vi "Actuator Channel Names DAO.vi"(5 "section":string="Auto Balance Error", 7 "Config Ref  In":T3, 8 "error in (no error)":errorcluster, 9 "Names In":T2, 10 "LBCB Number":T1, 11 "Actions":T4) -> (0 "error out":errorcluster, 1 "Names Out":T2, 6 "Config Ref Out":T3)   [LabVIEW 2009]
uses:
  Metadata/Persistant DAO Actions.ctl
  Metadata/Actuator Channel Names.ctl
  <vilib>/Utility/config.llb/Config Data RefNum.ctl
  Metadata/LBCB Number.ctl
  <vilib>/Utility/config.llb/NI_LVConfig.lvlib
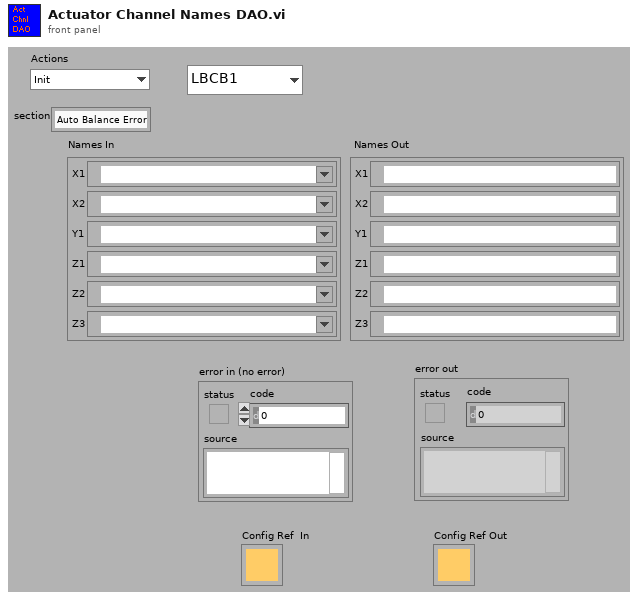
[diagram p1: front panel]
types:
  T1 = typedef "LBCB Number.ctl" = enum16{"LBCB1", "LBCB2"}
  T2 = typedef "Actuator Channel Names.ctl" = cluster{"X1":refnum<k21>, "X2":refnum<k21>, "Y1":refnum<k21>, "Z1":refnum<k21>, "Z2":refnum<k21>, "Z3":refnum<k21>}
  T3 = typedef "NI_LVConfig.lvlib/Config Data RefNum.ctl" = refnum<k1>
  T4 = typedef "Persistant DAO Actions.ctl" = enum16{"Init", "Get", "Set", "Load", "Save"}
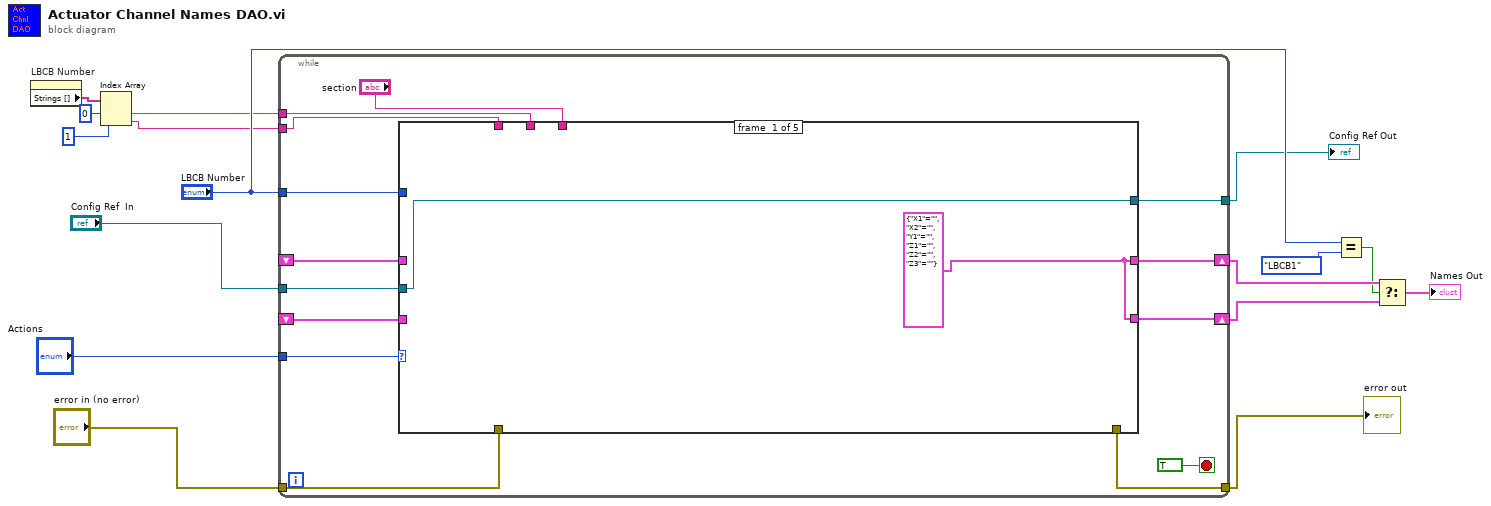
[diagram p0: block diagram]
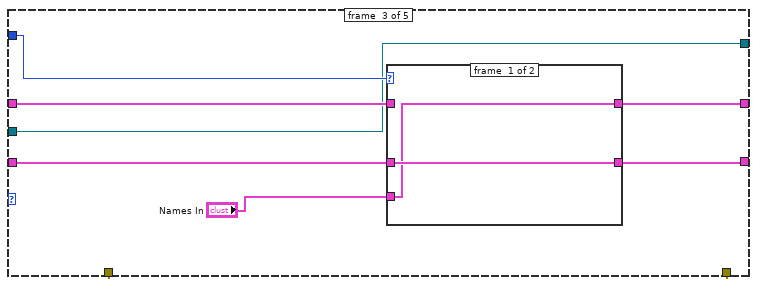
[diagram p3: hidden frame]
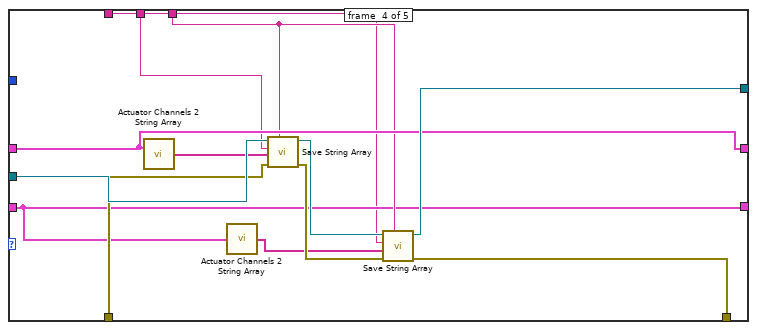
[diagram p5: hidden frame]
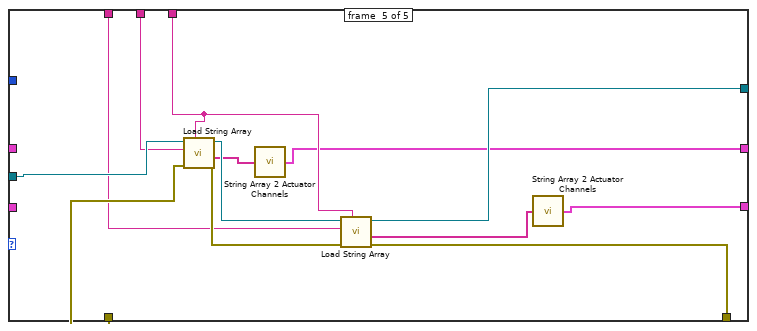
[diagram p6: hidden frame]
diagram:
  n1 = property on="LBCB Number" class="Enum (strict)"() -> ("Strings []"=w5:string[])  [unwired: 2 in, 2 out]
  n2 = Index Array(array=w5, index #1=0 ("index"), index #2=1 ("index")) -> (element #1=w2:string, element #2=w1:string)
  n3 = while {
    tunnel: "Actions" -> [w29]
    tunnel: "Config Ref  In" -> [w28]
    tunnel: "error in (no error)" -> [w26]
    tunnel: [w25] -> w6
    tunnel: [w24] -> w7
    shift-right: [w23] -> w13
    shift-left: _ -> [w22]
    tunnel: "LBCB Number" -> [w21]
    shift-right: [w20] -> w12
    shift-left: _ -> [w19]
    tunnel: w2 -> [w18]
    tunnel: w1 -> [w17]
    stop <- TRUE stop-if-true
    n4 = case shown="\"Load\"" w29 {
      tunnel: "section" -> [_ _ _ w54 w69]
      tunnel: w28 -> [w33 w35 w39 w62 w75]
      tunnel: w26 -> [w32 w34 w38 w61 w74]
      tunnel: [w33 w35 w39 w58 w71] -> w25
      tunnel: [w32 w34 w38 w57 w70] -> w24
      tunnel: [w31 w37 w40 w56 w63] -> w23
      tunnel: w22 -> [_ w37 w44 w56 _]
      tunnel: w21 -> [_ _ w45 _ _]
      tunnel: [w31 w36 w41 w53 w65] -> w20
      tunnel: w19 -> [_ w36 w43 w53 _]
      tunnel: w18 -> [_ _ _ w51 w68]
      tunnel: w17 -> [_ _ _ w50 w67]
      frame #0 {
        w31 = T2 {"X1"="", "X2"="", "Y1"="", "Z1"="", "Z2"="", "Z3"=""} ("Names In")
        (unwired) T2 {"X1"="", "X2"="", "Y1"="", "Z1"="", "Z2"="", "Z3"=""} ("Names In")
      }
      frame #1 {
      }
      frame #2 {
        n5 = case shown="\"LBCB2\"" w45 {
          tunnel: w44 -> [_ w49]
          tunnel: w43 -> [w47 _]
          tunnel: "Names In" -> [w46 w48]
          tunnel: [w46 w49] -> w40
          tunnel: [w47 w48] -> w41
          frame #0 {
          }
          frame #1 {
          }
        }
      }
      frame #3 {
        n6 = call "Actuator Channels 2 String Array.vi"("Actuator Channels"=w56) -> ("Array"=w55:string[])
        n7 = call "Actuator Channels 2 String Array.vi"("Actuator Channels"=w53) -> ("Array"=w52:string[])
        n8 = call "Save String Array.vi"("section"=w54, "error in (no error)"=w61, "String Array In"=w55, "key"=w51, "refnum"=w62) -> ("error out"=w60:errorcluster, "refnum out"=w59:T3)  [unwired: 1 in, 4 out]
        n9 = call "Save String Array.vi"("section"=w54, "error in (no error)"=w60, "String Array In"=w52, "key"=w50, "refnum"=w59) -> ("error out"=w57:errorcluster, "refnum out"=w58:T3)  [unwired: 1 in, 4 out]
      }
      frame #4 {
        n10 = call "Load String Array.vi"("section"=w69, "error in (no error)"=w74, "key"=w68, "refnum"=w75) -> ("error out"=w72:errorcluster, "String Array Out"=w64:string[], "refnum out"=w73:T3)  [unwired: 5 out]
        n11 = call "String Array 2 Actuator Channels.vi"("Array"=w64) -> ("Actuator Point"=w63:T2)
        n12 = call "Load String Array.vi"("section"=w69, "error in (no error)"=w72, "key"=w67, "refnum"=w73) -> ("error out"=w70:errorcluster, "String Array Out"=w66:string[], "refnum out"=w71:T3)  [unwired: 5 out]
        n13 = call "String Array 2 Actuator Channels.vi"("Array"=w66) -> ("Actuator Point"=w65:T2)
      }
    }
  }
  "error out" <- w7
  "Config Ref Out" <- w6
  n14 = Equal?(x="LBCB Number", y=LBCB_Number."LBCB1") -> (x = y?=w11:bool)
  n15 = Select(t=w13, s=w11, f=w12) -> (s? t:f=→"Names Out":T2)
